vi "PH_AWG-510.Evt Call Get Trigger Settings.vi"(0 "i ref in":refnum<vi>, 1 "Instance":string, 5 "error in":errorcluster) -> (14 "i ref out":refnum<vi>, 19 "error out":errorcluster)   [LabVIEW 2014, in "PH_AWG-510.lvlib"]
doc: "This VI calls a method by a simple call."
uses:
  PH_AWG-510.lvlib
  CS_Core/BaseProcess/BaseProcess.lvlib
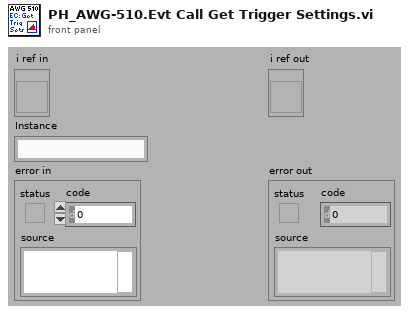
[diagram p1: front panel]
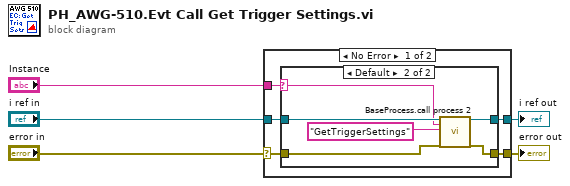
[diagram p0: block diagram]
diagram:
  n1 = case shown="No Error" "error in" {
    selector: "error in" -> [w7 w19]
    tunnel: [w10 w19] -> w2
    tunnel: "Instance" -> [w6 _]
    tunnel: "i ref in" -> [w9 w20]
    tunnel: [w8 w20] -> w4
    frame No Error {
      n2 = case shown="Default" w6 {
        selector: w6 -> [_ w13]
        tunnel: [w12 w18] -> w10
        tunnel: w7 -> [w12 w16]
        tunnel: w9 -> [w11 w15]
        tunnel: [w11 w14] -> w8
        frame "", "N/A" {
        }
        frame Default {
          n3 = call "BaseProcess.call process 2.vi"("i ref in"=w15, "Object"=w13, "Selector"="GetTriggerSettings", "error in (no error)"=w16) -> ("i ref out"=w14:refnum<vi>, "error out"=w18:errorcluster)  [unwired: 14 in]
        }
      }
    }
    frame Error {
    }
  }
  "i ref out" <- w4
  "error out" <- w2
